vi "CANOpen_Main_SDO parallel.vi"(8 "error in (no error)":errorcluster, 9 "SDO Asynch":T1 {"HW Dyn Read"."Resp Chan."."Chan Refs" format="%.0x"; "HW Dyn Read"."Req Chan."."Chan Refs" format="%.0x"; "HW Dyn Write"."Resp Chan."."Chan Refs" format="%.0x"; "HW Dyn Write"."Req Chan."."Chan Refs" format="%.0x"; "List SDO"."Resp Chan."."Chan Refs" format="%.0x"; "List SDO"."Req Chan."."Chan Refs" format="%.0x"}, 10 "SDO queues":T3, 11 "interface object in":refnum<k20>) -> (0 "error out":errorcluster)   [LabVIEW 2013, in "CANOpen Addon Custom Device.lvlib"]
uses:
  CANOpen Addon Custom Device.lvlib
  CanOpen_SDO queue ref.ctl
  SDO queue.ctl
  Shared Code/CANOpen_SDO Settings.ctl
  SubVIS/CANOpen_VS SDOs Data Refs.ctl
  <vilib>/NI Veristand/Custom Device API/Data Reference.ctl
  CanOpen_SDO Dynamic queue.ctl
  Shared Code/CANOpen_SDO queue W data.ctl
  Shared Code/CANOpen_SDO queue mode.ctl
  Shared Code/CANOpen_PDO Data Type in queue.ctl
  <vilib>/NI Veristand/Custom Device API/Custom Device Timed Loop Priority.ctl
  <vilib>/Platform/TimedLoop/XDataNode/timing_clust.ctl
  <vilib>/Platform/TimedLoop/XDataNode/nitl_modes.ctl
  <vilib>/Platform/TimedLoop/XDataNode/wakeup.ctl
  <vilib>/CANopenLib/CANOPEN.llb/CANopen SDO Close.vi
  <vilib>/CANopenLib/CANOPEN.llb/CANopen SDO Write [Block].vi
  <vilib>/CANopenLib/CANOPEN.llb/CANopen SDO Create.vi
  <vilib>/CANopenLib/CANOPEN.llb/CANopen SDO Write [I8].vi
  <vilib>/CANopenLib/CANOPEN.llb/CANopen SDO Write [I16].vi
  <vilib>/CANopenLib/CANOPEN.llb/CANopen SDO Write [I32].vi
  <vilib>/CANopenLib/CANOPEN.llb/CANopen SDO Write [SGL].vi
  <vilib>/CANopenLib/CANOPEN.llb/CANopen SDO Write [DBL].vi
  <vilib>/CANopenLib/CANOPEN.llb/CANopen SDO Write [U16].vi
  <vilib>/CANopenLib/CANOPEN.llb/CANopen SDO Write [U32].vi
  <vilib>/CANopenLib/CANOPEN.llb/CANopen SDO Write [U8].vi
  <vilib>/CANopenLib/CANOPEN.llb/CANopen SDO Read [U16].vi
  <vilib>/CANopenLib/CANOPEN.llb/CANopen SDO Read [U32].vi
  <vilib>/CANopenLib/CANOPEN.llb/CANopen SDO Read [I16].vi
  <vilib>/CANopenLib/CANOPEN.llb/CANopen SDO Read [I32].vi
  <vilib>/CANopenLib/CANOPEN.llb/CANopen SDO Read [SGL].vi
  <vilib>/CANopenLib/CANOPEN.llb/CANopen SDO Read [DBL].vi
  <vilib>/CANopenLib/CANOPEN.llb/CANopen SDO Read [I8].vi
  <vilib>/CANopenLib/CANOPEN.llb/CANopen SDO Read [U8].vi
  <vilib>/Platform/TimedLoop/XDataNode/XDataNode.xnode
  <vilib>/NI Veristand/Custom Device API/Custom Device API.lvlib
  <vilib>/Platform/TimedLoop/XDataNode/XDNodeRunTimeDep.lvlib
panel:
  # "LSB"
  # "MSB"
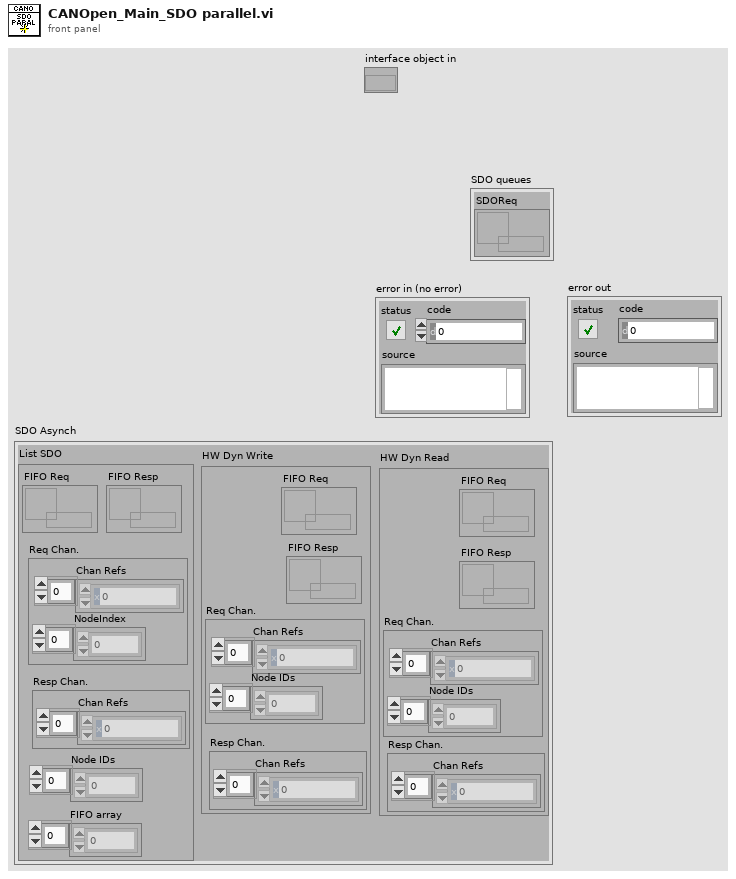
[diagram p1: front panel]
types:
  T1 = typedef "CANOpen Addon Custom Device.lvlib/CANOpen_VS SDOs Data Refs.ctl" = cluster{"List SDO":cluster{"FIFO Req":refnum<k33>, "Req Chan.":cluster{"Chan Refs":T2[], "NodeIndex":dbl[]}, "FIFO Resp":refnum<k33>, "Resp Chan.":cluster{"Chan Refs":T2[]}, "Node IDs":u8[], "FIFO array":dbl[]}, "HW Dyn Write":cluster{"FIFO Req":refnum<k33>, "FIFO Resp":refnum<k33>, "Req Chan.":cluster{"Chan Refs":T2[], "Node IDs":u8[]}, "Resp Chan.":cluster{"Chan Refs":T2[]}}, "HW Dyn Read":cluster{"FIFO Req":refnum<k33>, "FIFO Resp":refnum<k33>, "Req Chan.":cluster{"Chan Refs":T2[], "Node IDs":u8[]}, "Resp Chan.":cluster{"Chan Refs":T2[]}}}
  T2 = typedef "Custom Device API.lvlib/Data Reference.ctl" = i32
  T3 = typedef "CANOpen Addon Custom Device.lvlib/CanOpen_SDO queue ref.ctl" = cluster{"SDOReq":refnum<queue>}
  T4 = typedef "Custom Device API.lvlib/Custom Device Timed Loop Priority.ctl" = enum32{"Low", "Medium", "High"}
  T5 = typedef "XDNodeRunTimeDep.lvlib/timing_clust.ctl" = cluster{"Expected End [f-1]":u64, "Actual End [f-1]":u64, "Finished Late? [f-1]":bool, "Expected End [i-1]":u64, "Actual End [i-1]":u64, "Finished Late? [i-1]":bool, "Expected Start [i]":u64, "Actual Start [i]":u64, "Expected Start [f]":u64, "Actual Start [f]":u64, "Source Name":string, "Structure Name":string, "Period":i64, "Deadline":i64, "Offset":i64, "Start":i64, "Priority":i32, "Timeout":i32, "Mode":T6, "Wakeup Reason":T7, "Error":errorcluster, "Source Type":string, "Secondary Source Type":string, "Global End Time":u64, "Global Start Time":u64, "Frame Duration":u64, "Iteration Duration":u64, "Assigned CPU":i32, "I/O Scan Engine Mode":u32}
  T6 = typedef "XDNodeRunTimeDep.lvlib/nitl_modes.ctl" = enum32{"No Change", "Process missed periods, maintain original phase", "Discard missed periods, maintain original phase", "Process missed periods, ignore original phase", "Discard missed periods, ignore original phase"}
  T7 = typedef "XDNodeRunTimeDep.lvlib/wakeup.ctl" = enum32{"Normal", "Aborted", "Asynchronous wakeup", "Timing source error", "Timed loop error", "Timeout"}
  T8 = typedef "CANOpen Addon Custom Device.lvlib/CANOpen_SDO queue mode.ctl" = enum16{"WRITE write", "WRITE response", "READ write", "READ response"}
  T9 = typedef "CANOpen Addon Custom Device.lvlib/CANOpen_PDO Data Type in queue.ctl" = enum16{"U8", "U16", "U32", "I8", "I16", "I32", "Single", "Double"}
  T10 = typedef "CANOpen Addon Custom Device.lvlib/CanOpen_SDO Dynamic queue.ctl" = cluster{"Node ID":u8, "Data":T11}
  T11 = typedef "CANOpen Addon Custom Device.lvlib/CANOpen_SDO queue W data.ctl" = cluster{"Object Index":u16, "Object Sub-Index (0)":u8, "Mode":T8, "Data Type":T9, "Value":dbl, "Status code":dbl, "Byte Order":enum16{"big-endian, network order", "little-endian"}}
  T12 = enum16{"big-endian, network order", "native, host order", "little-endian"}
  T13 = typedef "CANOpen Addon Custom Device.lvlib/SDO queue.ctl" = cluster{"element":T14, "Node ID":u8}
  T14 = typedef "CANOpen Addon Custom Device.lvlib/CANOpen_SDO Settings.ctl" = cluster{"Object Index":u16, "Sub-Index (0)":u8, "Block Data":u8[], "Name":string}
  T15 = enum16{"big-endian, network order", "little-endian"}
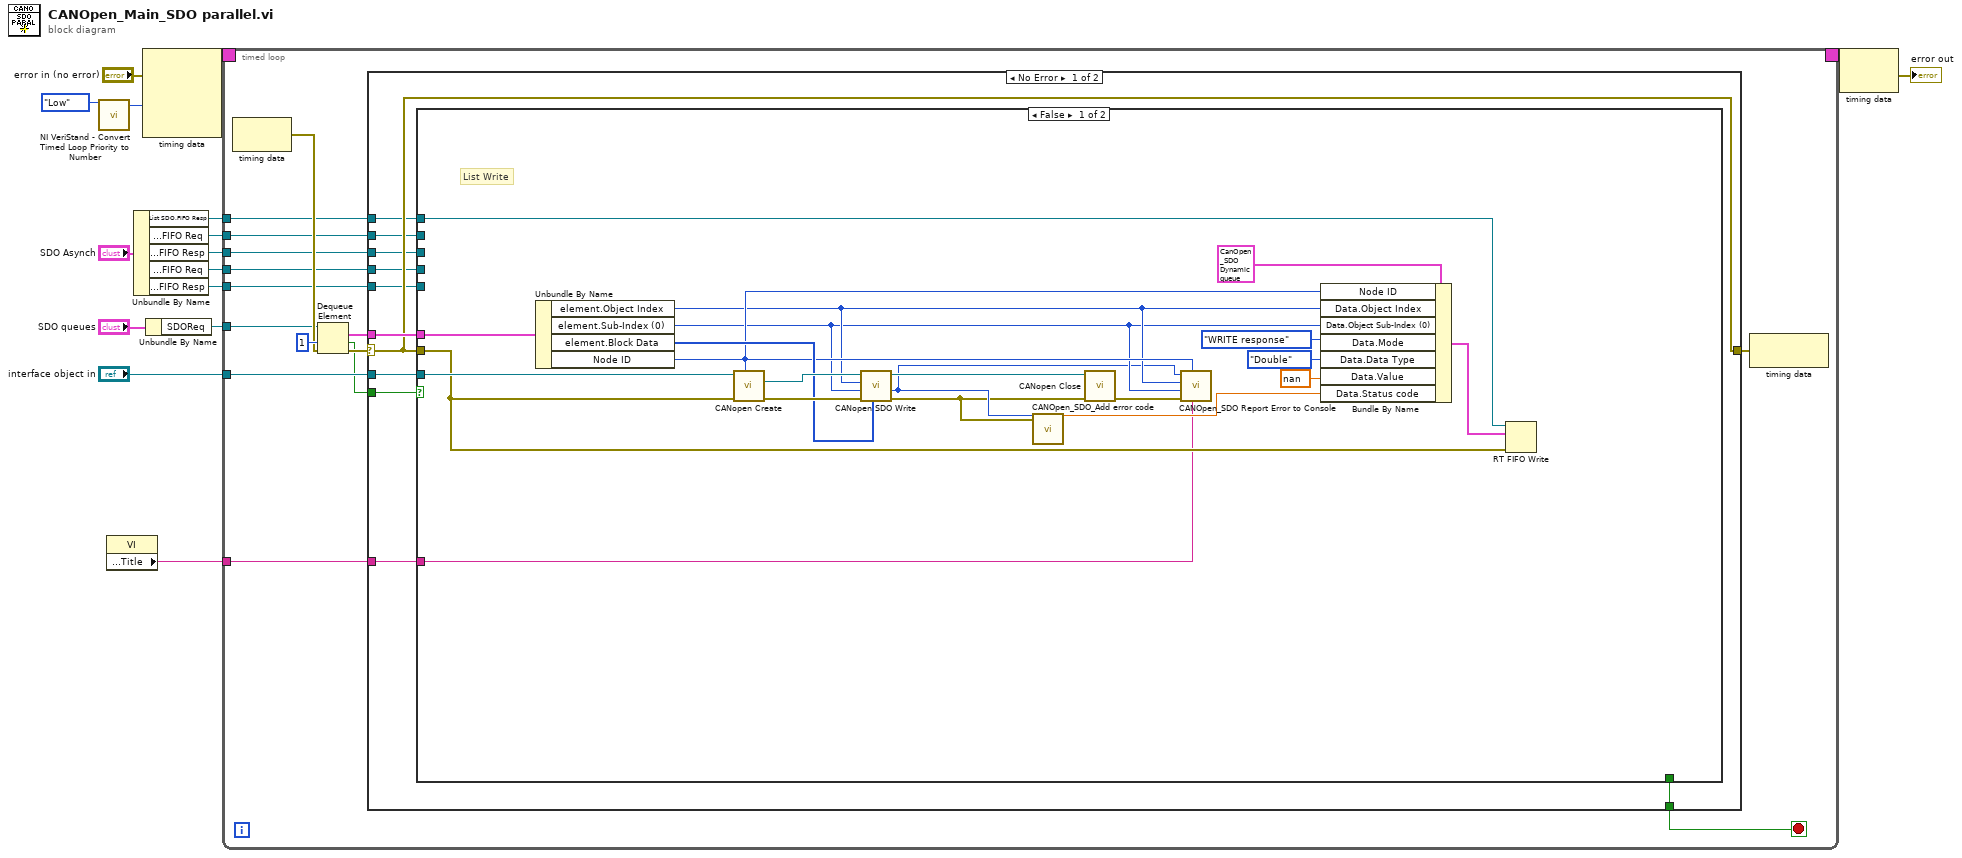
[diagram p0: block diagram]
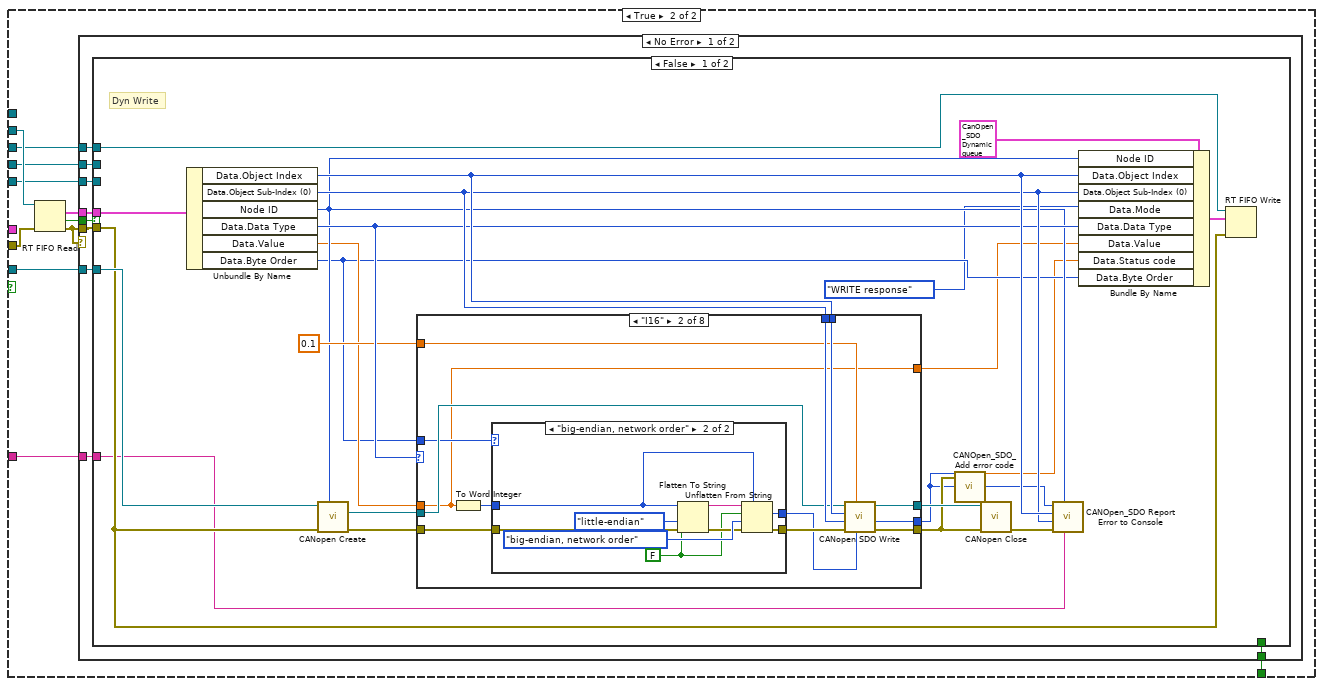
[diagram p2: hidden frame]
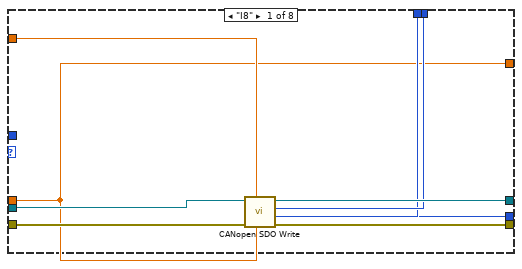
[diagram p3: hidden frame]
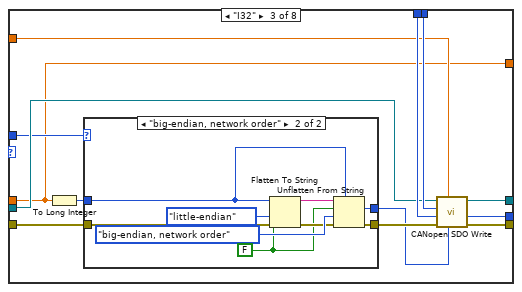
[diagram p5: hidden frame]
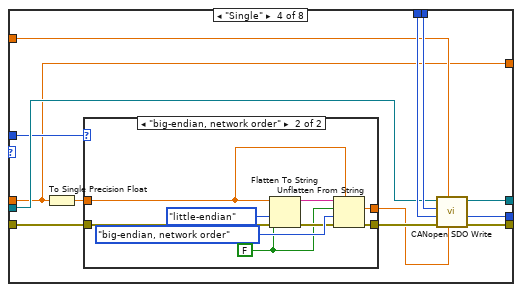
[diagram p7: hidden frame]
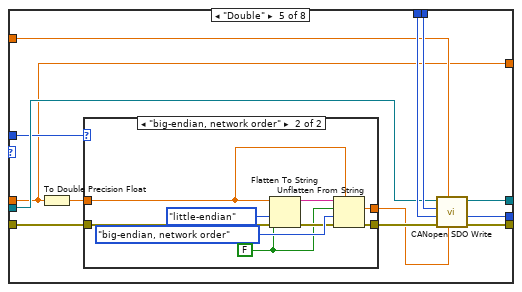
[diagram p9: hidden frame]
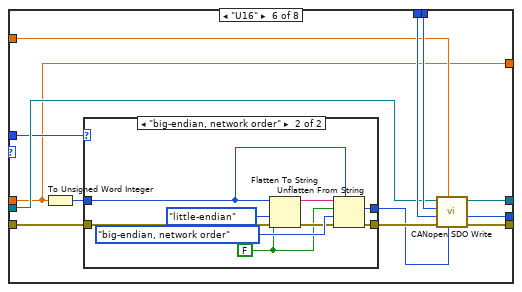
[diagram p11: hidden frame]
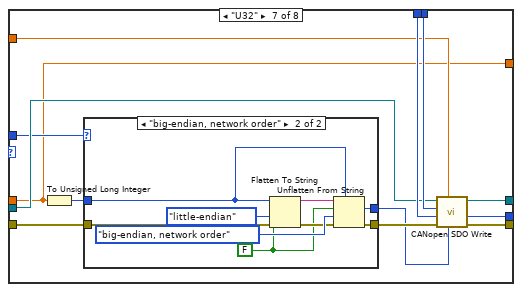
[diagram p13: hidden frame]
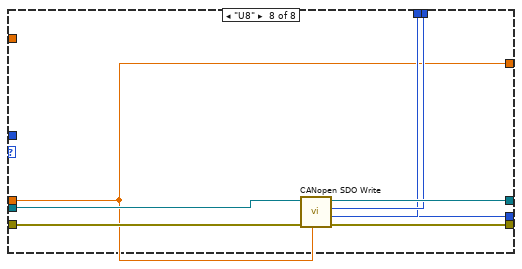
[diagram p15: hidden frame]
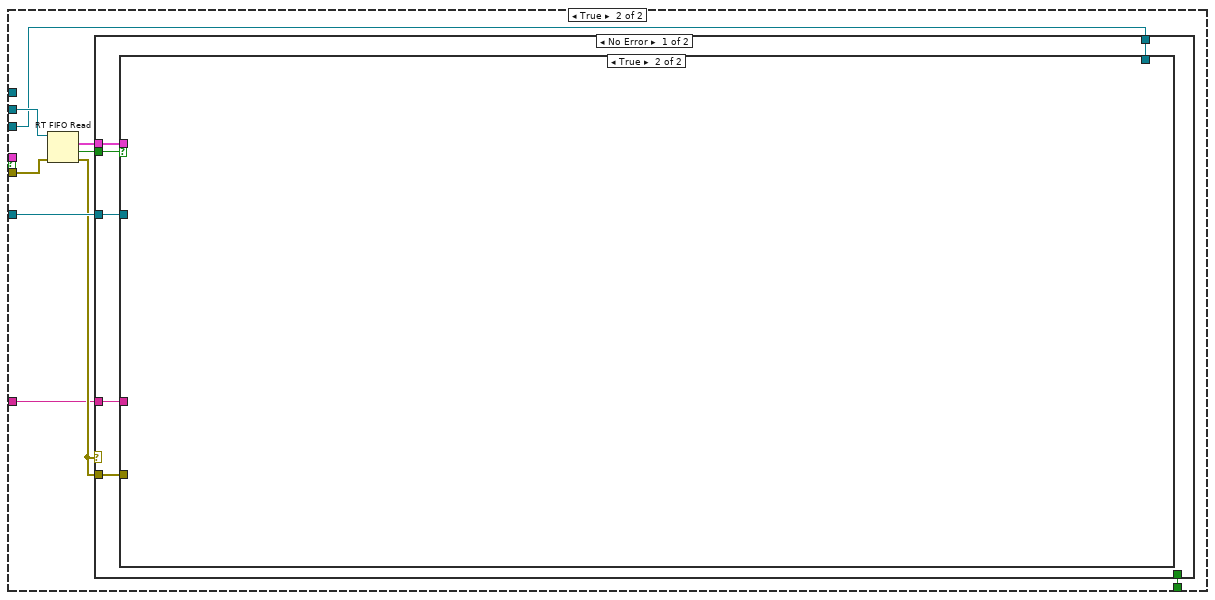
[diagram p16: hidden frame]
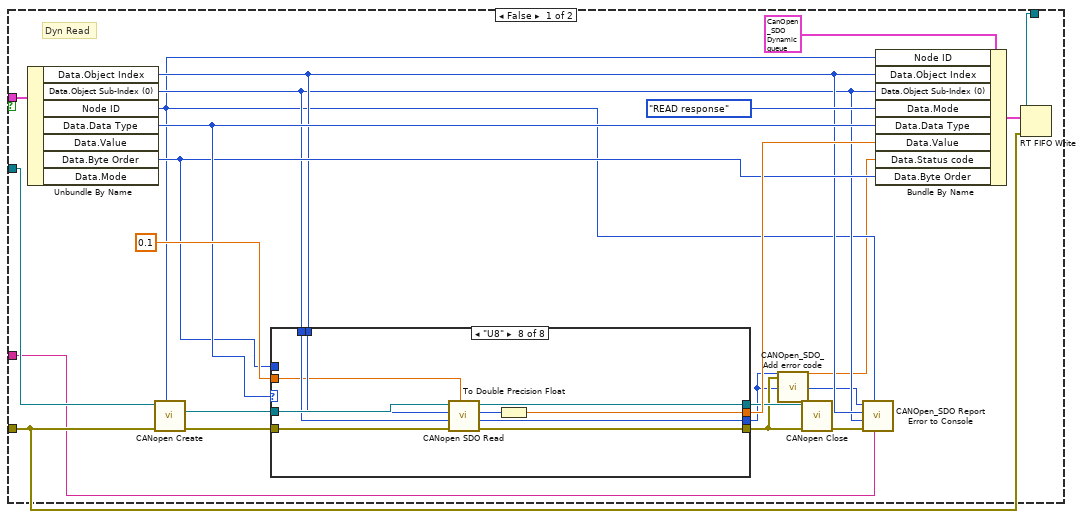
[diagram p17: hidden frame]
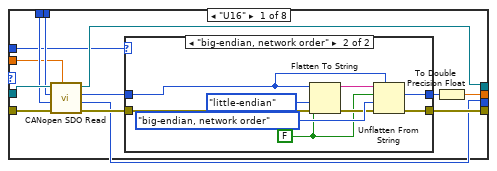
[diagram p18: hidden frame]
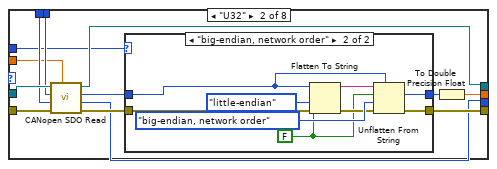
[diagram p20: hidden frame]
diagram:
  n1 = call <vilib>:"NI VeriStand - Convert Timed Loop Priority to Number.vi"("Priority"=Custom_Device_Timed_Loop_Priority."Low") -> ("Numeric Priority"=w12:i32)  [unwired: 10 in]
  n2 = property class="VI"() -> ("Front Panel.Title"=w1:string)  [unwired: 2 in, 2 out]
  n3 = Unbundle By Name("SDO Asynch") -> ("List SDO.FIFO Resp"=w6:refnum<k33>, "HW Dyn Write.FIFO Req"=w5:refnum<k33>, "HW Dyn Write.FIFO Resp"=w4:refnum<k33>, "HW Dyn Read.FIFO Req"=w3:refnum<k33>, "HW Dyn Read.FIFO Resp"=w2:refnum<k33>)
  n4 = node-c288("error in (no error)", w12) -> (w14:T5)  [unwired: 2 in]
  n5 = Unbundle By Name("SDO queues") -> ("SDOReq"=w8:refnum<queue>)
  n6 = timed-loop {
    tunnel: "interface object in" -> [w28]
    timing: w14 -> [_]
    timing-out: [_] -> w13
    tunnel: w8 -> [w23]
    tunnel: w6 -> [w22]
    tunnel: w5 -> [w21]
    tunnel: w4 -> [w20]
    tunnel: w3 -> [w19]
    tunnel: w2 -> [w18]
    tunnel: w1 -> [w17]
    stop <- w30 stop-if-true
    n7 = node-c288() -> (w24:errorcluster)  [unwired: 1 in]
    n8 = Dequeue Element(queue=w23, timeout in ms (-1)=1, error in (no error)=w24) -> (element=w29:T13, timed out?=w26:bool, error out=w31:errorcluster)  [unwired: 1 out]
    n9 = case shown="No Error" w31 {
      selector: w31 -> [w45 _]
      tunnel: [w38 TRUE] -> w30
      tunnel: w29 -> [w47 _]
      tunnel: w28 -> [w46 _]
      tunnel: [w45 errorcluster {"status"=FALSE, "code"=0, "source"=""} ("error out")] -> w25
      tunnel: w26 -> [w44 _]
      tunnel: w22 -> [w43 _]
      tunnel: w21 -> [w42 _]
      tunnel: w20 -> [w41 _]
      tunnel: w19 -> [w40 _]
      tunnel: w18 -> [w39 _]
      tunnel: w17 -> [w37 _]
      frame No Error {
        n10 = case shown="False" w44 {
          tunnel: w47 -> [w68 _]
          tunnel: w46 -> [w64 w76]
          tunnel: w45 -> [w61 w78]
          tunnel: w43 -> [w52 _]
          tunnel: w42 -> [_ w75]
          tunnel: w41 -> [_ w74]
          tunnel: w40 -> [_ w73]
          tunnel: w39 -> [_ w72]
          tunnel: [_ w70] -> w38
          tunnel: w37 -> [w48 w69]
          frame False {
            # "List Write"
            n11 = Unbundle By Name(w68) -> ("element.Object Index"=w57:u16, "element.Sub-Index (0)"=w56:u8, "element.Block Data"=w63:u8[], "Node ID"=w58:u8)
            n12 = call-poly <vilib>:"CANopen Create.vi"("node-ID"=w58, "error in (no error)"=w61, "interface object in"=w64) -> ("error out"=w66:errorcluster, "SDO object out"=w65:refnum<k20>)  [unwired: 6 in, 1 out]
            n13 = call-poly <vilib>:"CANopen SDO Write.vi"("block data"=w63, "error in (no error)"=w66, "object sub-index (0)"=w56, "object index"=w57, "SDO object in"=w65) -> ("error out"=w49:errorcluster, "completion code"=w50:u32, "SDO object out"=w67:refnum<k20>)  [unwired: 4 in]
            n14 = call "CANOpen_SDO_Add error code.vi"("completion code in"=w50, "error in (no error)"=w49) -> ("completion code out"=w51:dbl)  [unwired: 25 in]
            n15 = call-poly <vilib>:"CANopen Close.vi"("error in (no error)"=w49, "SDO object in"=w67) -> ("error out"=w62:errorcluster)  [unwired: 9 in]
            n16 = call "CANOpen_SDO Report Error to Console.vi"("Caller"=w48, "Node ID"=w58, "error in (no error)"=w62, "Object Sub-Index"=w56, "Object Index"=w57, "completion code"=w50) -> ()  [unwired: 6 in]
            n17 = Bundle By Name(cluster=T10 {"Node ID"=0, "Data"={"Object Index"=0, "Object Sub-Index (0)"=0, "Mode"=enum."WRITE response", "Data Type"=enum."Double", "Value"=0.0, "Status code"=0.0, "Byte Order"=enum."big-endian, network order"}} ("element"), "Node ID"=w58, "Data.Object Index"=w57, "Data.Object Sub-Index (0)"=w56, "Data.Mode"=CANOpen_SDO_queue_mode."WRITE response", "Data.Data Type"=CANOpen_PDO_Data_Type_in_queue."Double", "Data.Value"=nan, "Data.Status code"=w51) -> (w59:T10)
            n18 = RT FIFO Write(0:w52, 1:w59, 3:w61) -> ()  [unwired: 2 in, 4 out]
          }
          frame True {
            n19 = RT FIFO Read(0:w75, 3:w78) -> (9:w77:T10, 10:w79:bool, 11:w71:errorcluster)  [unwired: 2 in, 2 out]
            n20 = case shown="No Error" w71 {
              tunnel: w79 -> [w88 _]
              tunnel: w71 -> [w87 _]
              tunnel: w77 -> [w86 _]
              tunnel: w76 -> [w85 _]
              tunnel: w74 -> [w84 _]
              tunnel: w73 -> [w83 _]
              tunnel: w72 -> [w82 _]
              tunnel: [w81 TRUE] -> w70
              tunnel: w69 -> [w80 _]
              frame No Error {
                n21 = case shown="False" w88 {
                  tunnel: w87 -> [w98 w280]
                  tunnel: w86 -> [w106 _]
                  tunnel: w85 -> [w107 w281]
                  tunnel: w84 -> [w93 _]
                  tunnel: w83 -> [_ w277]
                  tunnel: w82 -> [_ w276]
                  tunnel: [_ w274] -> w81
                  tunnel: w80 -> [w89 w273]
                  frame False {
                    # "Dyn Write"
                    n22 = Unbundle By Name(w106) -> ("Data.Object Index"=w103:u16, "Data.Object Sub-Index (0)"=w102:u8, "Node ID"=w99:u8, "Data.Data Type"=w101:T9, "Data.Value"=w97:dbl, "Data.Byte Order"=w96:T15)
                    n23 = call-poly <vilib>:"CANopen Create.vi"("node-ID"=w99, "error in (no error)"=w98, "interface object in"=w107) -> ("error out"=w110:errorcluster, "SDO object out"=w109:refnum<k20>)  [unwired: 6 in, 1 out]
                    n24 = case shown="\"I16\"" w101 {
                      tunnel: [w120 w133 w157 w181 w205 w229 w253 w272] -> w92
                      tunnel: [w119 w132 w156 w180 w204 w228 w252 w271] -> w111
                      tunnel: w110 -> [w118 w127 w151 w175 w199 w223 w247 w270]
                      tunnel: w109 -> [w117 w125 w149 w173 w197 w221 w245 w269]
                      tunnel: w103 -> [w116 w131 w155 w179 w203 w227 w251 w268]
                      tunnel: w102 -> [w115 w130 w154 w178 w202 w226 w250 w267]
                      tunnel: [w114 w129 w153 w177 w201 w225 w249 w266] -> w90
                      tunnel: 0.1 ("timeout (1s)") -> [w113 w128 w152 w176 w200 w224 w248 _]
                      tunnel: w97 -> [w112 w121 w145 w169 w193 w217 w241 w265]
                      tunnel: w96 -> [_ w122 w147 w171 w195 w219 w243 _]
                      tunnel: [w112 w121 w145 w169 w193 w217 w241 w265] -> w95
                      frame "I8" {
                        n25 = call-poly <vilib>:"CANopen SDO Write.vi"("I8 data"=w112, "timeout (1s)"=w113, "error in (no error)"=w118, "object sub-index (0)"=w115, "object index"=w116, "SDO object in"=w117) -> ("error out"=w120:errorcluster, "completion code"=w114:u32, "SDO object out"=w119:refnum<k20>)  [unwired: 3 in]
                      }
                      frame "I16" {
                        n26 = To Word Integer(number=w121) -> (16bit integer=w123:i16)
                        n27 = case shown="\"big-endian, network order\"" w122 {
                          tunnel: [w134 w140] -> w124
                          tunnel: w127 -> [w135 w139]
                          tunnel: [w135 w138] -> w126
                          tunnel: w123 -> [w134 w136]
                          frame "little-endian", Default {
                          }
                          frame "big-endian, network order" {
                            w137 = FALSE ("prepend array or string size? (T)")
                            n28 = Flatten To String(anything=w136, prepend array or string size? (T)=w137, byte order (0:big-endian, network order)=T12."little-endian", error in (no error)=w139) -> (data string=w143:string, error out=w141:errorcluster)  [unwired: 1 out]
                            n29 = Unflatten From String(type=w136, binary string=w143, data includes array or string size? (T)=w137, byte order (0:big-endian, network order)=T12."big-endian, network order", error in (no error)=w141) -> (value=w140:i16, error out=w138:errorcluster)  [unwired: 1 out]
                          }
                        }
                        n30 = call-poly <vilib>:"CANopen SDO Write.vi"("I16 data"=w124, "timeout (1s)"=w128, "error in (no error)"=w126, "object sub-index (0)"=w130, "object index"=w131, "SDO object in"=w125) -> ("error out"=w133:errorcluster, "completion code"=w129:u32, "SDO object out"=w132:refnum<k20>)  [unwired: 3 in]
                      }
                      frame "I32" {
                        n31 = To Long Integer(number=w145) -> (32bit integer=w146:i32)
                        n32 = case shown="\"big-endian, network order\"" w147 {
                          tunnel: [w158 w164] -> w148
                          tunnel: w151 -> [w159 w163]
                          tunnel: [w159 w162] -> w150
                          tunnel: w146 -> [w158 w160]
                          frame "little-endian", Default {
                          }
                          frame "big-endian, network order" {
                            w161 = FALSE ("prepend array or string size? (T)")
                            n33 = Flatten To String(anything=w160, prepend array or string size? (T)=w161, byte order (0:big-endian, network order)=T12."little-endian", error in (no error)=w163) -> (data string=w167:string, error out=w165:errorcluster)  [unwired: 1 out]
                            n34 = Unflatten From String(type=w160, binary string=w167, data includes array or string size? (T)=w161, byte order (0:big-endian, network order)=T12."big-endian, network order", error in (no error)=w165) -> (value=w164:i32, error out=w162:errorcluster)  [unwired: 1 out]
                          }
                        }
                        n35 = call-poly <vilib>:"CANopen SDO Write.vi"("I32 data"=w148, "timeout (1s)"=w152, "error in (no error)"=w150, "object sub-index (0)"=w154, "object index"=w155, "SDO object in"=w149) -> ("error out"=w157:errorcluster, "completion code"=w153:u32, "SDO object out"=w156:refnum<k20>)  [unwired: 3 in]
                      }
                      frame "Single" {
                        n36 = To Single Precision Float(number=w169) -> (single precision float=w170:sgl)
                        n37 = case shown="\"big-endian, network order\"" w171 {
                          tunnel: [w182 w188] -> w172
                          tunnel: w175 -> [w183 w187]
                          tunnel: [w183 w186] -> w174
                          tunnel: w170 -> [w182 w184]
                          frame "little-endian", Default {
                          }
                          frame "big-endian, network order" {
                            w185 = FALSE ("prepend array or string size? (T)")
                            n38 = Flatten To String(anything=w184, prepend array or string size? (T)=w185, byte order (0:big-endian, network order)=T12."little-endian", error in (no error)=w187) -> (data string=w191:string, error out=w189:errorcluster)  [unwired: 1 out]
                            n39 = Unflatten From String(type=w184, binary string=w191, data includes array or string size? (T)=w185, byte order (0:big-endian, network order)=T12."big-endian, network order", error in (no error)=w189) -> (value=w188:sgl, error out=w186:errorcluster)  [unwired: 1 out]
                          }
                        }
                        n40 = call-poly <vilib>:"CANopen SDO Write.vi"("SGL data"=w172, "timeout (1s)"=w176, "error in (no error)"=w174, "object sub-index (0)"=w178, "object index"=w179, "SDO object in"=w173) -> ("error out"=w181:errorcluster, "completion code"=w177:u32, "SDO object out"=w180:refnum<k20>)  [unwired: 3 in]
                      }
                      frame "Double" {
                        n41 = To Double Precision Float(number=w193) -> (double precision float=w194:dbl)
                        n42 = case shown="\"big-endian, network order\"" w195 {
                          tunnel: [w206 w212] -> w196
                          tunnel: w199 -> [w207 w211]
                          tunnel: [w207 w210] -> w198
                          tunnel: w194 -> [w206 w208]
                          frame "little-endian", Default {
                          }
                          frame "big-endian, network order" {
                            w209 = FALSE ("prepend array or string size? (T)")
                            n43 = Flatten To String(anything=w208, prepend array or string size? (T)=w209, byte order (0:big-endian, network order)=T12."little-endian", error in (no error)=w211) -> (data string=w215:string, error out=w213:errorcluster)  [unwired: 1 out]
                            n44 = Unflatten From String(type=w208, binary string=w215, data includes array or string size? (T)=w209, byte order (0:big-endian, network order)=T12."big-endian, network order", error in (no error)=w213) -> (value=w212:dbl, error out=w210:errorcluster)  [unwired: 1 out]
                          }
                        }
                        n45 = call-poly <vilib>:"CANopen SDO Write.vi"("DBL data"=w196, "timeout (1s)"=w200, "error in (no error)"=w198, "object sub-index (0)"=w202, "object index"=w203, "SDO object in"=w197) -> ("error out"=w205:errorcluster, "completion code"=w201:u32, "SDO object out"=w204:refnum<k20>)  [unwired: 3 in]
                      }
                      frame "U16" {
                        n46 = To Unsigned Word Integer(number=w217) -> (unsigned 16bit integer=w218:u16)
                        n47 = case shown="\"big-endian, network order\"" w219 {
                          tunnel: [w230 w236] -> w220
                          tunnel: w223 -> [w231 w235]
                          tunnel: [w231 w234] -> w222
                          tunnel: w218 -> [w230 w232]
                          frame "little-endian", Default {
                          }
                          frame "big-endian, network order" {
                            w233 = FALSE ("prepend array or string size? (T)")
                            n48 = Flatten To String(anything=w232, prepend array or string size? (T)=w233, byte order (0:big-endian, network order)=T12."little-endian", error in (no error)=w235) -> (data string=w239:string, error out=w237:errorcluster)  [unwired: 1 out]
                            n49 = Unflatten From String(type=w232, binary string=w239, data includes array or string size? (T)=w233, byte order (0:big-endian, network order)=T12."big-endian, network order", error in (no error)=w237) -> (value=w236:u16, error out=w234:errorcluster)  [unwired: 1 out]
                          }
                        }
                        n50 = call-poly <vilib>:"CANopen SDO Write.vi"("U16 data"=w220, "timeout (1s)"=w224, "error in (no error)"=w222, "object sub-index (0)"=w226, "object index"=w227, "SDO object in"=w221) -> ("error out"=w229:errorcluster, "completion code"=w225:u32, "SDO object out"=w228:refnum<k20>)  [unwired: 3 in]
                      }
                      frame "U32" {
                        n51 = To Unsigned Long Integer(number=w241) -> (unsigned 32bit integer=w242:u32)
                        n52 = case shown="\"big-endian, network order\"" w243 {
                          tunnel: [w254 w260] -> w244
                          tunnel: w247 -> [w255 w259]
                          tunnel: [w255 w258] -> w246
                          tunnel: w242 -> [w254 w256]
                          frame "little-endian", Default {
                          }
                          frame "big-endian, network order" {
                            w257 = FALSE ("prepend array or string size? (T)")
                            n53 = Flatten To String(anything=w256, prepend array or string size? (T)=w257, byte order (0:big-endian, network order)=T12."little-endian", error in (no error)=w259) -> (data string=w263:string, error out=w261:errorcluster)  [unwired: 1 out]
                            n54 = Unflatten From String(type=w256, binary string=w263, data includes array or string size? (T)=w257, byte order (0:big-endian, network order)=T12."big-endian, network order", error in (no error)=w261) -> (value=w260:u32, error out=w258:errorcluster)  [unwired: 1 out]
                          }
                        }
                        n55 = call-poly <vilib>:"CANopen SDO Write.vi"("U32 data"=w244, "timeout (1s)"=w248, "error in (no error)"=w246, "object sub-index (0)"=w250, "object index"=w251, "SDO object in"=w245) -> ("error out"=w253:errorcluster, "completion code"=w249:u32, "SDO object out"=w252:refnum<k20>)  [unwired: 3 in]
                      }
                      frame "U8" {
                        n56 = call-poly <vilib>:"CANopen SDO Write.vi"("U8 data"=w265, "error in (no error)"=w270, "object sub-index (0)"=w267, "object index"=w268, "SDO object in"=w269) -> ("error out"=w272:errorcluster, "completion code"=w266:u32, "SDO object out"=w271:refnum<k20>)  [unwired: 4 in]
                      }
                    }
                    n57 = call "CANOpen_SDO_Add error code.vi"("completion code in"=w90, "error in (no error)"=w92) -> ("completion code out"=w91:dbl)  [unwired: 25 in]
                    n58 = call-poly <vilib>:"CANopen Close.vi"("error in (no error)"=w92, "SDO object in"=w111) -> ("error out"=w108:errorcluster)  [unwired: 9 in]
                    n59 = call "CANOpen_SDO Report Error to Console.vi"("Caller"=w89, "Node ID"=w99, "error in (no error)"=w108, "Object Sub-Index"=w102, "Object Index"=w103, "completion code"=w90) -> ()  [unwired: 6 in]
                    n60 = Bundle By Name(cluster=T10 {"Node ID"=0, "Data"={"Object Index"=0, "Object Sub-Index (0)"=0, "Mode"=enum."WRITE response", "Data Type"=enum."Double", "Value"=0.0, "Status code"=0.0, "Byte Order"=enum."big-endian, network order"}} ("element"), "Node ID"=w99, "Data.Object Index"=w103, "Data.Object Sub-Index (0)"=w102, "Data.Mode"=CANOpen_SDO_queue_mode."WRITE response", "Data.Data Type"=w101, "Data.Value"=w95, "Data.Status code"=w91, "Data.Byte Order"=w96) -> (w104:T10)
                    n61 = RT FIFO Write(0:w93, 1:w104, 3:w98) -> ()  [unwired: 2 in, 4 out]
                  }
                  frame True {
                    n62 = RT FIFO Read(0:w277, 3:w280) -> (9:w278:T10, 10:w279:bool, 11:w275:errorcluster)  [unwired: 2 in, 2 out]
                    n63 = case shown="No Error" w275 {
                      tunnel: w281 -> [w287 _]
                      tunnel: w275 -> [w286 _]
                      tunnel: w279 -> [w285 _]
                      tunnel: w278 -> [w284 _]
                      tunnel: w276 -> [w283 _]
                      tunnel: [_ TRUE] -> w274
                      tunnel: w273 -> [w282 _]
                      frame No Error {
                        n64 = case shown="True" w285 {
                          tunnel: w287 -> [w308 _]
                          tunnel: w286 -> [w295 _]
                          tunnel: w284 -> [w294 _]
                          tunnel: w283 -> [w292 _]
                          tunnel: w282 -> [w288 _]
                          frame False {
                            # "Dyn Read"
                            n65 = Unbundle By Name(w294) -> ("Data.Object Index"=w297:u16, "Data.Object Sub-Index (0)"=w296:u8, "Node ID"=w293:u8, "Data.Data Type"=w299:T9, "Data.Byte Order"=w298:T15)  [unwired: 2 out]
                            n66 = call-poly <vilib>:"CANopen Create.vi"("node-ID"=w293, "error in (no error)"=w295, "interface object in"=w308) -> ("error out"=w300:errorcluster, "SDO object out"=w301:refnum<k20>)  [unwired: 6 in, 1 out]
                            n67 = case shown="\"U8\"" w299 {
                              tunnel: [w313 w337 w361 w385 w409 w433 w463 w473] -> w291
                              tunnel: [w312 w336 w360 w384 w408 w432 w462 w472] -> w303
                              tunnel: w300 -> [w322 w346 w370 w394 w418 w442 w461 w471]
                              tunnel: w301 -> [w321 w345 w369 w393 w417 w441 w460 w470]
                              tunnel: w297 -> [w320 w344 w368 w392 w416 w440 w459 w469]
                              tunnel: w296 -> [w319 w343 w367 w391 w415 w439 w458 w468]
                              tunnel: [w311 w335 w359 w383 w407 w431 w457 w467] -> w289
                              tunnel: 0.1 ("timeout (1s)") -> [w318 w342 w366 w390 w414 w438 w456 w466]
                              tunnel: [w317 w341 w365 w389 w413 w437 w454 w464] -> w304
                              tunnel: w298 -> [w310 w334 w358 w382 w406 w430 _ _]
                              frame "U16" {
                                n68 = call-poly <vilib>:"CANopen SDO Read.vi"("timeout (1s)"=w318, "error in (no error)"=w322, "object sub-index (0)"=w319, "object index"=w320, "SDO object in"=w321) -> ("error out"=w315:errorcluster, "completion code"=w311:u32, "U16 data"=w316:u16, "SDO object out"=w312:refnum<k20>)  [unwired: 3 in]
                                n69 = case shown="\"big-endian, network order\"" w310 {
                                tunnel: w316 -> [w323 w329]
                                tunnel: [w323 w328] -> w314
                                tunnel: w315 -> [w324 w327]
                                tunnel: [w324 w326] -> w313
                                frame "little-endian", Default {
                                }
                                frame "big-endian, network order" {
                                w325 = FALSE ("prepend array or string size? (T)")
                                n70 = Flatten To String(anything=w329, prepend array or string size? (T)=w325, byte order (0:big-endian, network order)=T12."little-endian", error in (no error)=w327) -> (data string=w332:string, error out=w330:errorcluster)  [unwired: 1 out]
                                n71 = Unflatten From String(type=w329, binary string=w332, data includes array or string size? (T)=w325, byte order (0:big-endian, network order)=T12."big-endian, network order", error in (no error)=w330) -> (value=w328:u16, error out=w326:errorcluster)  [unwired: 1 out]
                                }
                                }
                                n72 = To Double Precision Float(number=w314) -> (double precision float=w317:dbl)
                              }
                              frame "U32" {
                                n73 = call-poly <vilib>:"CANopen SDO Read.vi"("timeout (1s)"=w342, "error in (no error)"=w346, "object sub-index (0)"=w343, "object index"=w344, "SDO object in"=w345) -> ("error out"=w339:errorcluster, "completion code"=w335:u32, "U32 data"=w340:u32, "SDO object out"=w336:refnum<k20>)  [unwired: 3 in]
                                n74 = case shown="\"big-endian, network order\"" w334 {
                                tunnel: w340 -> [w347 w353]
                                tunnel: [w347 w352] -> w338
                                tunnel: w339 -> [w348 w351]
                                tunnel: [w348 w350] -> w337
                                frame "little-endian", Default {
                                }
                                frame "big-endian, network order" {
                                w349 = FALSE ("prepend array or string size? (T)")
                                n75 = Flatten To String(anything=w353, prepend array or string size? (T)=w349, byte order (0:big-endian, network order)=T12."little-endian", error in (no error)=w351) -> (data string=w356:string, error out=w354:errorcluster)  [unwired: 1 out]
                                n76 = Unflatten From String(type=w353, binary string=w356, data includes array or string size? (T)=w349, byte order (0:big-endian, network order)=T12."big-endian, network order", error in (no error)=w354) -> (value=w352:u32, error out=w350:errorcluster)  [unwired: 1 out]
                                }
                                }
                                n77 = To Double Precision Float(number=w338) -> (double precision float=w341:dbl)
                              }
                              frame "I16" {
                                n78 = call-poly <vilib>:"CANopen SDO Read.vi"("timeout (1s)"=w366, "error in (no error)"=w370, "object sub-index (0)"=w367, "object index"=w368, "SDO object in"=w369) -> ("error out"=w363:errorcluster, "completion code"=w359:u32, "I16 data"=w364:i16, "SDO object out"=w360:refnum<k20>)  [unwired: 3 in]
                                n79 = case shown="\"big-endian, network order\"" w358 {
                                tunnel: w364 -> [w371 w377]
                                tunnel: [w371 w376] -> w362
                                tunnel: w363 -> [w372 w375]
                                tunnel: [w372 w374] -> w361
                                frame "little-endian", Default {
                                }
                                frame "big-endian, network order" {
                                w373 = FALSE ("prepend array or string size? (T)")
                                n80 = Flatten To String(anything=w377, prepend array or string size? (T)=w373, byte order (0:big-endian, network order)=T12."little-endian", error in (no error)=w375) -> (data string=w380:string, error out=w378:errorcluster)  [unwired: 1 out]
                                n81 = Unflatten From String(type=w377, binary string=w380, data includes array or string size? (T)=w373, byte order (0:big-endian, network order)=T12."big-endian, network order", error in (no error)=w378) -> (value=w376:i16, error out=w374:errorcluster)  [unwired: 1 out]
                                }
                                }
                                n82 = To Double Precision Float(number=w362) -> (double precision float=w365:dbl)
                              }
                              frame "I32" {
                                n83 = call-poly <vilib>:"CANopen SDO Read.vi"("timeout (1s)"=w390, "error in (no error)"=w394, "object sub-index (0)"=w391, "object index"=w392, "SDO object in"=w393) -> ("error out"=w387:errorcluster, "completion code"=w383:u32, "I32 data"=w388:i32, "SDO object out"=w384:refnum<k20>)  [unwired: 3 in]
                                n84 = case shown="\"big-endian, network order\"" w382 {
                                tunnel: w388 -> [w395 w401]
                                tunnel: [w395 w400] -> w386
                                tunnel: w387 -> [w396 w399]
                                tunnel: [w396 w398] -> w385
                                frame "little-endian", Default {
                                }
                                frame "big-endian, network order" {
                                w397 = FALSE ("prepend array or string size? (T)")
                                n85 = Flatten To String(anything=w401, prepend array or string size? (T)=w397, byte order (0:big-endian, network order)=T12."little-endian", error in (no error)=w399) -> (data string=w404:string, error out=w402:errorcluster)  [unwired: 1 out]
                                n86 = Unflatten From String(type=w401, binary string=w404, data includes array or string size? (T)=w397, byte order (0:big-endian, network order)=T12."big-endian, network order", error in (no error)=w402) -> (value=w400:i32, error out=w398:errorcluster)  [unwired: 1 out]
                                }
                                }
                                n87 = To Double Precision Float(number=w386) -> (double precision float=w389:dbl)
                              }
                              frame "Single" {
                                n88 = call-poly <vilib>:"CANopen SDO Read.vi"("timeout (1s)"=w414, "error in (no error)"=w418, "object sub-index (0)"=w415, "object index"=w416, "SDO object in"=w417) -> ("error out"=w411:errorcluster, "completion code"=w407:u32, "SGL data"=w412:sgl, "SDO object out"=w408:refnum<k20>)  [unwired: 3 in]
                                n89 = case shown="\"big-endian, network order\"" w406 {
                                tunnel: w412 -> [w419 w425]
                                tunnel: [w419 w424] -> w410
                                tunnel: w411 -> [w420 w423]
                                tunnel: [w420 w422] -> w409
                                frame "little-endian", Default {
                                }
                                frame "big-endian, network order" {
                                w421 = FALSE ("prepend array or string size? (T)")
                                n90 = Flatten To String(anything=w425, prepend array or string size? (T)=w421, byte order (0:big-endian, network order)=T12."little-endian", error in (no error)=w423) -> (data string=w428:string, error out=w426:errorcluster)  [unwired: 1 out]
                                n91 = Unflatten From String(type=w425, binary string=w428, data includes array or string size? (T)=w421, byte order (0:big-endian, network order)=T12."big-endian, network order", error in (no error)=w426) -> (value=w424:sgl, error out=w422:errorcluster)  [unwired: 1 out]
                                }
                                }
                                n92 = To Double Precision Float(number=w410) -> (double precision float=w413:dbl)
                              }
                              frame "Double" {
                                n93 = call-poly <vilib>:"CANopen SDO Read.vi"("timeout (1s)"=w438, "error in (no error)"=w442, "object sub-index (0)"=w439, "object index"=w440, "SDO object in"=w441) -> ("error out"=w435:errorcluster, "completion code"=w431:u32, "DBL data"=w436:dbl, "SDO object out"=w432:refnum<k20>)  [unwired: 3 in]
                                n94 = case shown="\"big-endian, network order\"" w430 {
                                tunnel: w436 -> [w443 w449]
                                tunnel: [w443 w448] -> w434
                                tunnel: w435 -> [w444 w447]
                                tunnel: [w444 w446] -> w433
                                frame "little-endian", Default {
                                }
                                frame "big-endian, network order" {
                                w445 = FALSE ("prepend array or string size? (T)")
                                n95 = Flatten To String(anything=w449, prepend array or string size? (T)=w445, byte order (0:big-endian, network order)=T12."little-endian", error in (no error)=w447) -> (data string=w452:string, error out=w450:errorcluster)  [unwired: 1 out]
                                n96 = Unflatten From String(type=w449, binary string=w452, data includes array or string size? (T)=w445, byte order (0:big-endian, network order)=T12."big-endian, network order", error in (no error)=w450) -> (value=w448:dbl, error out=w446:errorcluster)  [unwired: 1 out]
                                }
                                }
                                n97 = To Double Precision Float(number=w434) -> (double precision float=w437:dbl)
                              }
                              frame "I8" {
                                n98 = call-poly <vilib>:"CANopen SDO Read.vi"("timeout (1s)"=w456, "error in (no error)"=w461, "object sub-index (0)"=w458, "object index"=w459, "SDO object in"=w460) -> ("error out"=w463:errorcluster, "completion code"=w457:u32, "I8 data"=w455:i8, "SDO object out"=w462:refnum<k20>)  [unwired: 3 in]
                                n99 = To Double Precision Float(number=w455) -> (double precision float=w454:dbl)
                              }
                              frame "U8" {
                                n100 = call-poly <vilib>:"CANopen SDO Read.vi"("timeout (1s)"=w466, "error in (no error)"=w471, "object sub-index (0)"=w468, "object index"=w469, "SDO object in"=w470) -> ("error out"=w473:errorcluster, "completion code"=w467:u32, "U8 data"=w465:u8, "SDO object out"=w472:refnum<k20>)  [unwired: 3 in]
                                n101 = To Double Precision Float(number=w465) -> (double precision float=w464:dbl)
                              }
                            }
                            n102 = call "CANOpen_SDO_Add error code.vi"("completion code in"=w289, "error in (no error)"=w291) -> ("completion code out"=w290:dbl)  [unwired: 25 in]
                            n103 = call-poly <vilib>:"CANopen Close.vi"("error in (no error)"=w291, "SDO object in"=w303) -> ("error out"=w309:errorcluster)  [unwired: 9 in]
                            n104 = call "CANOpen_SDO Report Error to Console.vi"("Caller"=w288, "Node ID"=w293, "error in (no error)"=w309, "Object Sub-Index"=w296, "Object Index"=w297, "completion code"=w289) -> ()  [unwired: 6 in]
                            n105 = Bundle By Name(cluster=T10 {"Node ID"=0, "Data"={"Object Index"=0, "Object Sub-Index (0)"=0, "Mode"=enum."WRITE response", "Data Type"=enum."Double", "Value"=0.0, "Status code"=0.0, "Byte Order"=enum."big-endian, network order"}} ("element"), "Node ID"=w293, "Data.Object Index"=w297, "Data.Object Sub-Index (0)"=w296, "Data.Mode"=CANOpen_SDO_queue_mode."READ response", "Data.Data Type"=w299, "Data.Value"=w304, "Data.Status code"=w290, "Data.Byte Order"=w298) -> (w306:T10)
                            n106 = RT FIFO Write(0:w292, 1:w306, 3:w295) -> ()  [unwired: 2 in, 4 out]
                          }
                          frame True {
                          }
                        }
                      }
                      frame Error {
                      }
                    }
                  }
                }
              }
              frame Error {
              }
            }
          }
        }
      }
      frame Error {
      }
    }
    n107 = node-c288(w25) -> ()  [unwired: 1 out]
  }
  n108 = node-c288(w13) -> (→"error out":errorcluster)
